vi "Name.CheckErrors.NoID.vi"(7 "Existing Frames":string[](array[string]), 8 "error in (no error)":errorcluster, 11 "Name":string) -> (0 "error out":errorcluster, 2 "Error String":string, 3 "Error?":bool)   [LabVIEW 2019, in "Diagnostics Addon System Explorer.lvlib"]
uses:
  Diagnostics Addon System Explorer.lvlib
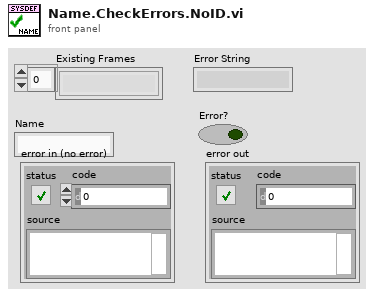
[diagram p1: front panel]
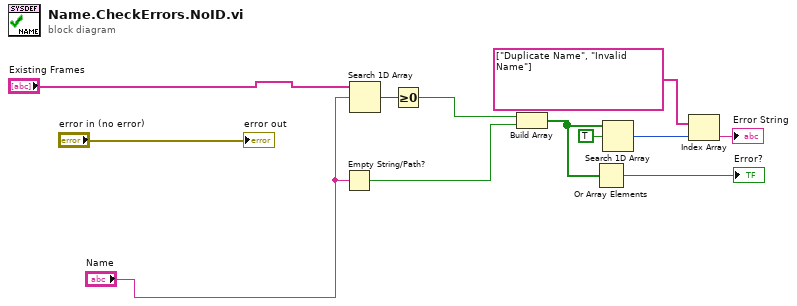
[diagram p0: block diagram]
diagram:
  n1 = Empty String/Path?(string/path="Name") -> (empty?=w4:bool)
  n2 = Search 1D Array(1D array="Existing Frames", element="Name") -> (index of element=w12:i32)  [unwired: 1 in]
  n3 = Greater Or Equal To 0?(x=w12) -> (x >= 0?=w5:bool)
  n4 = Build Array(w5, w4) -> (w9:bool[])
  n5 = Or Array Elements(Boolean array=w9) -> (logical OR=→"Error?":bool)
  n6 = Search 1D Array(1D array=w9, element=TRUE) -> (index of element=w7:i32)  [unwired: 1 in]
  n7 = Index Array(array=string[] ["Duplicate Name", "Invalid Name"], index=w7) -> (element=→"Error String":string)
  "error out" <- "error in (no error)"
